vi "Rate Limiter.vi"(9 "Initial Value":dbl, 10 "Limit":dbl, 11 "Value":dbl) -> (3 "Output":dbl)   [LabVIEW 2015]
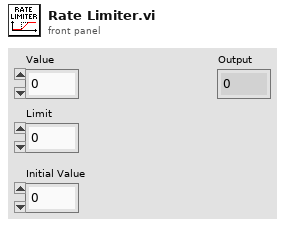
[diagram p1: front panel]
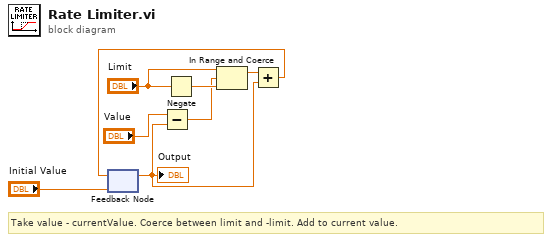
[diagram p0: block diagram]
diagram:
  # "Take value - currentValue. Coerce between limit and -limit. Add to current value."
  n1 = feedback #1("Initial Value") -> (w2:dbl)
  "Output" <- w2
  n2 = Subtract(x="Value", y=w2) -> (x-y=w6:dbl)
  n3 = Negate(x="Limit") -> (-x=w8:dbl)
  n4 = In Range and Coerce(upper limit="Limit", x=w6, lower limit=w8) -> (coerced(x)=w7:dbl)  [unwired: 1 out]
  n5 = Add(x=w7, y=w2) -> (x+y=w5:dbl)
  n6 = feedback-in #1(w5) -> ()
